vi "Test checkbox cell.vi"(11 "Test Case In":refnum<class "Test Cases.lvclass">) -> (0 "error out":errorcluster, 3 "Test Case Out":refnum<class "Test Cases.lvclass">)   [LabVIEW 2024, in "Test Cases.lvclass"]
uses:
  Test Cases.lvclass
  C:/Program Files/National Instruments/LabVIEW 2025/vi.lib/Astemes/LUnit/Test Case.lvclass
  D:/git/Sourcegrid-LabVIEW/dll/SourceGrid.dll
  dll/SourceGrid.dll
  source/Grid/SourceGrid.lvclass
  source/Cells/Check Box/Check Box.lvclass
  D:/git/Sourcegrid-LabVIEW/source/Cells/Cell/Cell.lvclass
  <vilib>/Astemes/LUnit/Test Case.lvclass/Test Case.ctl
  Test Cases.lvclass/Test Cases.ctl
  <vilib>/Astemes/LUnit/Test Case.lvclass
  D:/git/Sourcegrid-LabVIEW/source/Cells/Check Box/Check Box.lvclass
panel:
  in  "stop":bool
  in  "Grid Container":refnum<k24>(container)
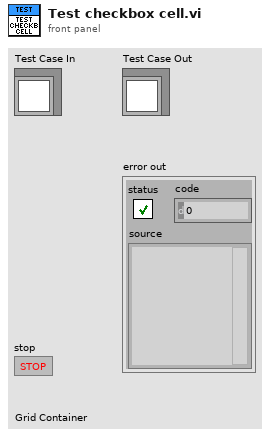
[diagram p1: front panel]
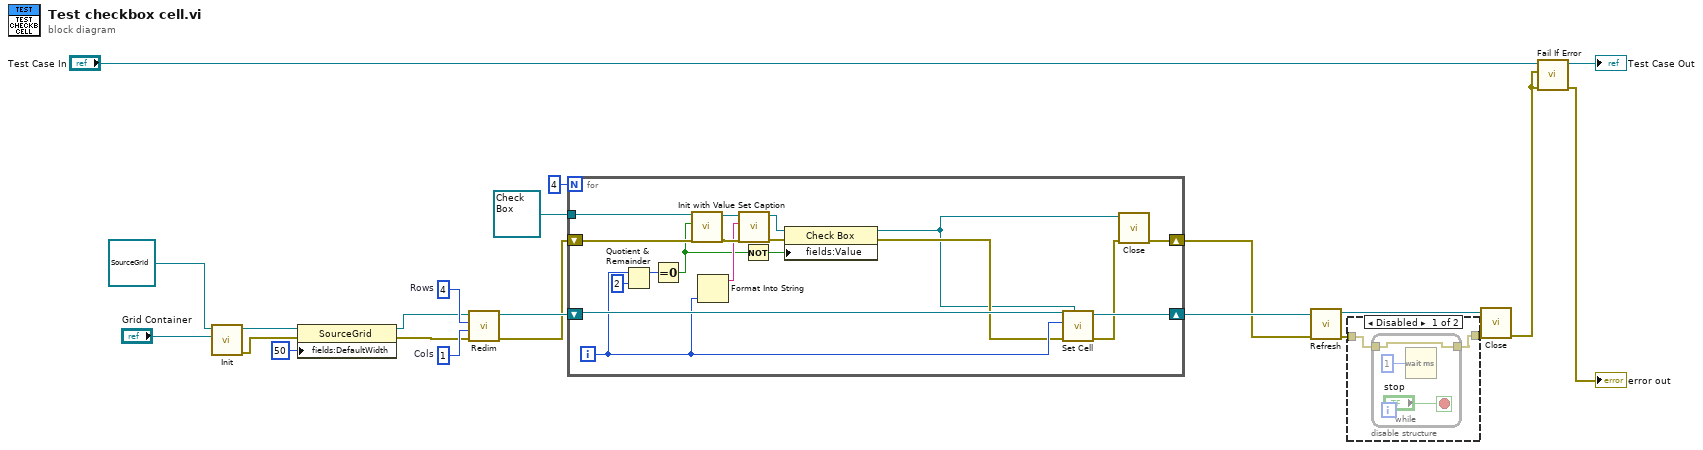
[diagram p0: block diagram]
diagram:
  w18 = 1  # Cols
  w19 = 4  # Rows
  n1 = call-dynamic "Init.vi"("Sourcegrid Container"="Grid Container", "Grid in"=refnum<class "SourceGrid.lvclass"> refnum) -> ("error out"=w6:errorcluster, "Grid out"=w15:refnum<class "SourceGrid.lvclass">)  [unwired: 8 in]
  n2 = property class="SourceGrid"(reference=w15, error in=w6, "fields:DefaultWidth"=50 ("DefaultWidth")) -> (reference out=w14:refnum<class "SourceGrid.lvclass">, error out=w13:errorcluster)
  n3 = call "Redim.vi"("error in"=w13, "Columns"=w18, "Rows"=w19, "Sourcegrid in"=w14) -> ("error out"=w1:errorcluster, "Sourcegrid out"=w10:refnum<class "SourceGrid.lvclass">)  [unwired: 6 in]
  n4 = for {
    N: 4 -> [_]
    shift-right: [w38] -> w2
    shift-left: w1 -> [w35]
    shift-right: [w40] -> w11
    shift-left: w10 -> [w39]
    tunnel: refnum<class "Check Box.lvclass"> refnum ("Cell in") -> [w36]
    i -> [w29]
    n5 = Quotient & Remainder(x=w29, y=2) -> (x-y*floor(x/y)=w32:i32)  [unwired: 1 out]
    n6 = Equal To 0?(x=w32) -> (x = 0?=w24:bool)
    n7 = call-dynamic "Init with Value.vi"("error in"=w35, "Value"=w24, "Check Box in"=w36) -> ("error out"=w34:errorcluster, "Check Box out"=w30:refnum<class "Check Box.lvclass">)  [unwired: 7 in]
    n8 = Format Into String(w29) -> (resulting string=w28:string)  [unwired: 3 in, 1 out]
    n9 = call-dynamic "Set Caption.vi"("error in"=w34, "Caption"=w28, "Check Box in"=w30) -> ("error out"=w31:errorcluster, "Check Box out"=w26:refnum<class "Check Box.lvclass">)  [unwired: 7 in]
    n10 = Not(x=w24) -> (.not. x?=w23:bool)
    n11 = property class="Check Box"(reference=w26, error in=w31, "fields:Value"=w23) -> (reference out=w25:refnum<class "Check Box.lvclass">, error out=w27:errorcluster)
    n12 = call "Set Cell.vi"("Cell"=w25, "error in"=w27, "Row"=w29, "Sourcegrid in"=w39) -> ("error out"=w37:errorcluster, "Sourcegrid out"=w40:refnum<class "SourceGrid.lvclass">)  [unwired: 6 in]
    n13 = call-dynamic "Close.vi"("error in"=w37, "Cell in"=w25) -> ("error out"=w38:errorcluster)  [unwired: 8 in, 1 out]
  }
  n14 = call "Refresh.vi"("error in"=w2, "SourceGrid in"=w11) -> ("error out"=w4:errorcluster, "SourceGrid out"=w8:refnum<class "SourceGrid.lvclass">)  [unwired: 8 in]
  n15 = disable-structure shown="Disabled" {
    disable-tunnel: w4 -> [w42 w46]
    disable-tunnel: [w41 w46] -> w3
    frame Disabled {
      n16 = while {
        tunnel: w42 -> [w43]
        tunnel: [w43] -> w41
        stop <- "stop" stop-if-true
        n17 = Wait (ms)(milliseconds to wait=u32 1) -> ()  [unwired: 1 out]
      }
    }
    frame Enabled {
    }
  }
  n18 = call-dynamic "Close.vi"("error in"=w3, "Sourcegrid in"=w8) -> ("error out"=w17:errorcluster)  [unwired: 8 in, 1 out]
  n19 = call <vilib>:"Fail If Error.vi"("error in (no error)"=w17, "Assert error"=w17, "LUnit Test Case In"="Test Case In") -> ("error out"=→"error out":errorcluster, "LUnit Test Case Out"=→"Test Case Out":refnum<class "Test Cases.lvclass">)  [unwired: 7 in]
